vi "Numeric_Integration.vi"() -> ()   [LabVIEW 2022 SP3]
uses:
  <vilib>/Analysis/8numeric.llb/1D Numeric Integration.vi
  <vilib>/Analysis/NI_AALPro.lvlib
panel:
  out "Percent Deviation":sgl format="%#_13e"
  out "Calculated Value":ext
  # "Numeric_Integration:\nThe program, once run, will calculate the \nintegral of (3x**2) from 0 to 1 using Simpson's\nMethod. This value as well as the percent deviation\nfrom the tru value will be shown below."
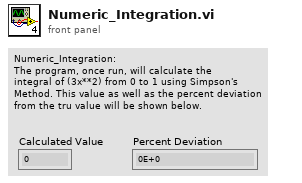
[diagram p1: front panel]
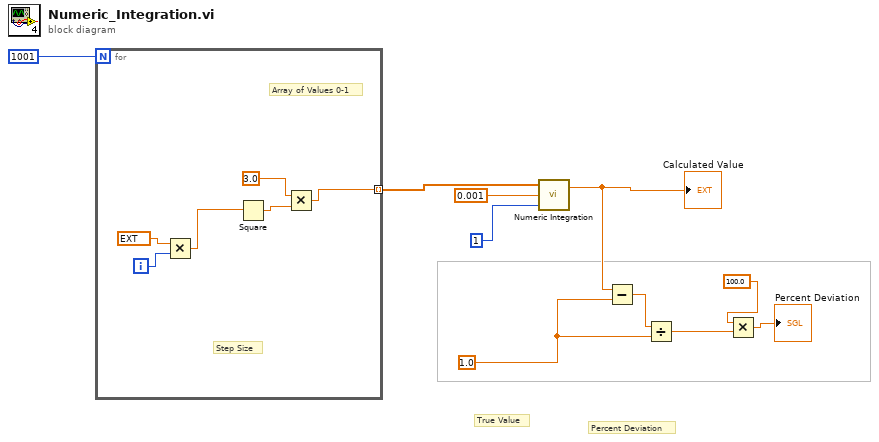
[diagram p0: block diagram]
diagram:
  w5 = 1.0
  # "True Value"
  # "Percent Deviation"
  n1 = for {
    N: 1001 -> [_]
    tunnel: [w11] -> w7 mode=indexing
    i -> [w15]
    # "Array of Values 0-1"
    # "Step Size"
    n2 = Multiply(x=ext 0.001, y=w15) -> (x*y=w12:ext)
    n3 = Square(x=w12) -> (x^2=w14:ext)
    n4 = Multiply(x=sgl 3.0, y=w14) -> (x*y=w11:ext)
  }
  n5 = call-poly <vilib>:"Numeric Integration.vi"("integration method"=1, "dt"=0.001, "Input Array"=w7) -> ("result"=w6:dbl)  [unwired: 1 out]
  "Calculated Value" <- w6
  n6 = Subtract(x=w6, y=w5) -> (x-y=w1:dbl)
  n7 = Divide(x=w1, y=w5) -> (x/y=w2:dbl)
  n8 = Multiply(x=sgl 100.0, y=w2) -> (x*y=→"Percent Deviation":dbl)
